vi "MAP.vi"(10 "input bit stream":i8[](array[numeric])) -> (2 "dout":cdb[](array[numeric]))   [LabVIEW 2010]
uses:
  <vilib>/addons/Modulation/Digital/Support/Controls/Pack Bits Parameters.ctl
  <vilib>/imath/engines/lvmath/Plug In/_Char/NIMS_CH_character datatype.ctl
  <vilib>/imath/engines/lvmath2/RunTimeEngine/ErrorHandling/NIMS_Finalize Error.vi
  <vilib>/imath/engines/lvmath2/RunTimeEngine/Managers/WorkSpace/UID Generator.vi
  <vilib>/imath/engines/lvmath2/RunTimeEngine/BuiltInFunctions/length/NIMS_length(GV).vi
  <instcachedir>/0/NIMS_length(GV)_08A3D13377FD4E4B96F5795FBF3698FA.lvgen/NIMS_length(GV)_08A3D13377FD4E4B96F5795FBF3698FA_002.vi
  <vilib>/imath/engines/lvmath2/RunTimeEngine/Managers/SymbolTable/Clear UID.vi
  <vilib>/imath/engines/lvmath2/RunTimeEngine/NodeEndStatement/NIMS_NodeEndStatement_Output.vi
  <instcachedir>/0/NIMS_NodeEndStatement_Output_53EC0D466D134D7ABD903AC30B43404B.lvgen/NIMS_NodeEndStatement_Output_53EC0D466D134D7ABD903AC30B43404B_000.vi
  <vilib>/imath/engines/lvmath2/RunTimeEngine/BuiltInFunctions/zeros/NIMS_V=zeros(I32,I32).vi
  <vilib>/imathl/engines/lvmath/Functions/Error Handling/Create Error.vi
  <vilib>/imath/engines/lvmath2/RunTimeEngine/RangeToken/NIMS_Range_R2 - Integer.vi
  <instcachedir>/0/NIMS_Range_R2 - Integer_217CA55F27D14E80B3D190635C7B3F47.lvgen/NIMS_Range_R2 - Integer_217CA55F27D14E80B3D190635C7B3F47_000.vi
  <vilib>/imath/engines/lvmath2/RunTimeEngine/CommandStatement/MC_CommandStatement_break.vi
  <vilib>/imath/engines/lvmath2/RunTimeEngine/VariableToken/Read/NIMS_Get Elements - RV(_) - Check.vi
  <instcachedir>/0/NIMS_Get Elements - RV(_) - Check_1F6F8656162345078B1D4DC9877DFAE9.lvgen/NIMS_Get Elements - RV(_) - Check_1F6F8656162345078B1D4DC9877DFAE9_004.vi
  <vilib>/imath/engines/lvmath2/RunTimeEngine/RunTimeType/NIMS_RunTimeType_From StrictType (excl LVString).vi
  <vilib>/imath/engines/lvmath2/RunTimeEngine/LocalVariableDefStatement/MC_LocalVariableDefStatement_Display.vi
  <vilib>/imath/engines/lvmath2/RunTimeEngine/ReplaceToken/NIMS_Replace - Check Linear.vi
  <instcachedir>/0/NIMS_Replace - Check Linear_662D5651E4E34E0584DA82A256193A4C.lvgen/NIMS_Replace - Check Linear_662D5651E4E34E0584DA82A256193A4C_002.vi
  <vilib>/imath/engines/lvmath2/RunTimeEngine/ReplaceToken/NIMS_Replace - Size Check _(_)=S.vi
  <instcachedir>/0/NIMS_Replace - Size Check _(_)=S_6CAC13ACC74349C582FDAB09BCDAB70F.lvgen/NIMS_Replace - Size Check _(_)=S_6CAC13ACC74349C582FDAB09BCDAB70F_001.vi
  <vilib>/imath/engines/lvmath2/RunTimeEngine/ReplaceToken/NIMS_Replace - V(S)=S.vi
  <instcachedir>/0/NIMS_Replace - V(S)=S_78FDB6CCD265407D8926E4CF958018EB.lvgen/NIMS_Replace - V(S)=S_78FDB6CCD265407D8926E4CF958018EB_001.vi
  <vilib>/addons/Modulation/niDMT.lvlib
  <vilib>/addons/Modulation/Digital/General/MT Generate Bits (Galois, PN Order).vi
  <vilib>/imath/engines/lvmath2/RunTimeEngine/Managers/SymbolTable/NIMS_WorkSpace.lvlib
panel:
  out "test":bool
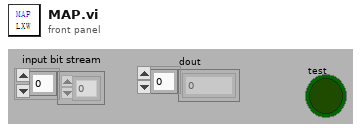
[diagram p1: front panel]
types:
  T1 = typedef "niDMT.lvlib/Pack Bits Parameters.ctl" = enum16{"Unsigned", "Signed"}
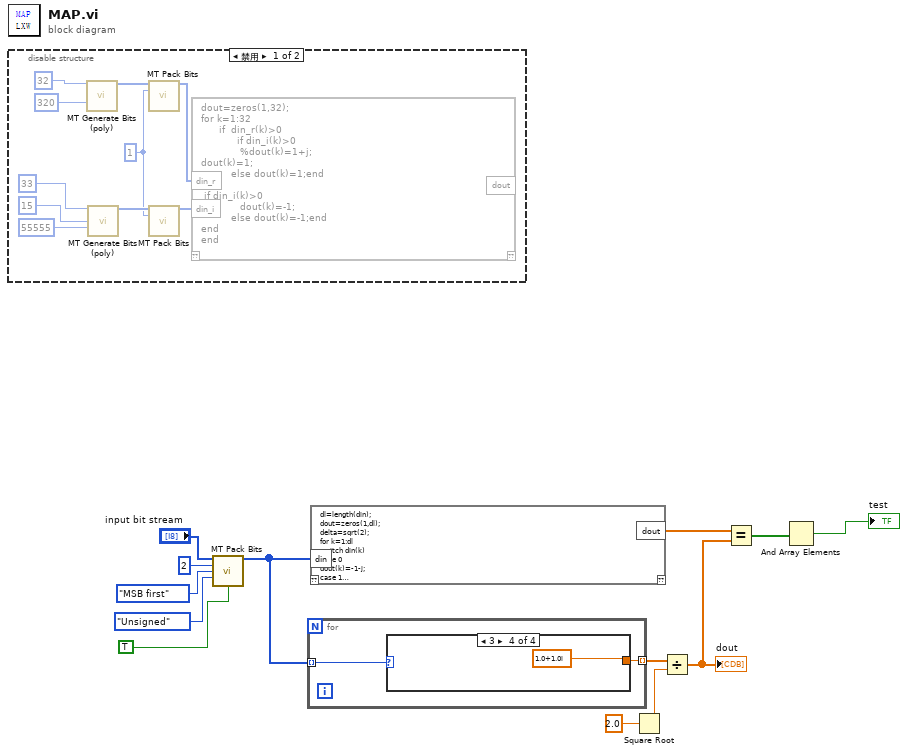
[diagram p0: block diagram]
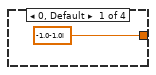
[diagram p2: hidden frame]
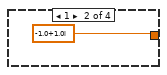
[diagram p3: hidden frame]
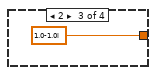
[diagram p4: hidden frame]
diagram:
  n1 = disable-structure shown="禁用" {
    frame Disabled {
      w17 = 1 ("bits per integer")
      n2 = call-poly <vilib>:"MT Generate Bits (poly).vi"("total bits (128)"=32, "seed in (0xD6BF7DF2)"=320) -> ("output bit stream"=w22:i8[])  [unwired: 11 in, 2 out]
      n3 = call-poly <vilib>:"MT Generate Bits (poly).vi"("total bits (128)"=33, "PN sequence order (9)"=15, "seed in (0xD6BF7DF2)"=55555) -> ("output bit stream"=w19:i8[])  [unwired: 10 in, 2 out]
      n4 = call <vilib>:"MT Pack Bits.vi"("input bit stream"=w22, "bits per integer"=w17) -> ("output integers"=w15:i32[])  [unwired: 12 in, 1 out]
      n5 = call <vilib>:"MT Pack Bits.vi"("input bit stream"=w19, "bits per integer"=w17) -> ("output integers"=w14:i32[])  [unwired: 12 in, 1 out]
      n6 = mathscript code="dout=zeros(1,32);\nfor k=1:32\n      if  din_r(k)>0\n            if din_i(k)>0\n             %dout(k)=1+j;\ndout(k)=1;\n          else dout(k)=1;end\nelse   \n if din_i(k)>0\n             dout(k)=-1;\n          else dout(k)=-1;end\nend\nend"("din_r"=w15, "din_i"=w14) -> ()  [unwired: 1 in, 2 out]
    }
    frame Enabled {
    }
  }
  n7 = call <vilib>:"MT Pack Bits.vi"("input bit stream"="input bit stream", "bits per integer"=2, "packed bit order"=enum16{"MSB first", "LSB first"}."MSB first", "integer format"=Pack_Bits_Parameters."Unsigned", "reset ? (T)"=TRUE) -> ("output integers"=w8:i32[])  [unwired: 9 in, 1 out]
  n8 = for {
    tunnel: w8 -> [w217] mode=indexing
    tunnel: [w216] -> w4 mode=indexing
    n9 = case shown="3" w217 {
      tunnel: [cdb -1.0-1.0i cdb -1.0+1.0i cdb 1.0-1.0i cdb 1.0+1.0i] -> w216
      frame 0, Default {
      }
      frame 1 {
      }
      frame 2 {
      }
      frame 3 {
      }
    }
  }
  n10 = mathscript code="dl=length(din);\ndout=zeros(1,dl);\ndelta=sqrt(2);\nfor k=1:dl\nswitch din(k)\ncase 0\ndout(k)=-1-j;\ncase 1\ndout(k)=-1+j;\ncase 2\ndout(k)=1-j;\ncase 3\ndout(k)=1+j;\notherwise\ndisp('Sorry,you are failed!!!!!!')\nend\nend\ndout=dout/delta;"("din"=w8) -> ("dout"=w7:cdb[])  [unwired: 1 in, 1 out]
  n11 = Square Root(x=2.0) -> (sqrt(x)=w2:dbl)
  n12 = Divide(x=w4, y=w2) -> (x/y=w1:cdb[])
  "dout" <- w1
  n13 = Equal?(x=w7, y=w1) -> (x = y?=w6:bool[])
  n14 = And Array Elements(Boolean array=w6) -> (logical AND=→"test":bool)
